vi "Example_External_File_Payload.vi"() -> ()   [LabVIEW 2020, in "PixPack.lvlib"]
uses:
  PixPack.lvlib
panel:
  out "error out":errorcluster
  in  "error in":errorcluster
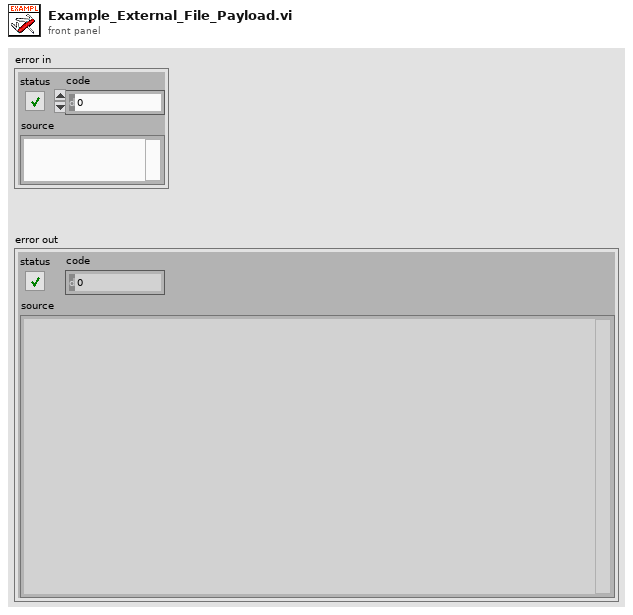
[diagram p1: front panel]
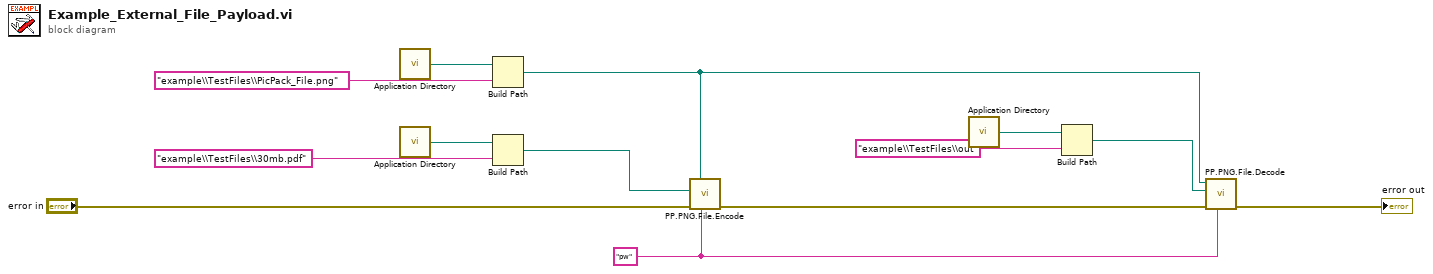
[diagram p0: block diagram]
diagram:
  w2 = "pw" ("Password")
  n1 = call <vilib>:"Application Directory.vi"() -> ("Application Directory"=w12:path)
  n2 = call <vilib>:"Application Directory.vi"() -> ("Application Directory"=w11:path)
  n3 = Build Path(base path=w12, name or relative path="example\\TestFiles\\PicPack_File.png") -> (appended path=w4:path)
  n4 = Build Path(base path=w11, name or relative path="example\\TestFiles\\30mb.pdf") -> (appended path=w6:path)
  n5 = call "PP.PNG.File.Encode.vi"("Password"=w2, "error in"="error in", "File Path"=w6, "PNG In"=w4) -> ("error out"=w5:errorcluster)  [unwired: 6 in]
  n6 = call <vilib>:"Application Directory.vi"() -> ("Application Directory"=w8:path)
  n7 = Build Path(base path=w8, name or relative path="example\\TestFiles\\out") -> (appended path=w3:path)
  n8 = call "PP.PNG.File.Decode.vi"("Password"=w2, "error in"=w5, "File Folder Out"=w3, "PNG In"=w4) -> ("error out"=→"error out":errorcluster)  [unwired: 6 in]
